vi "超标留样数据插入.vi"(0 "data输出":T1={"时间"=timestamp(3687928779.282504 s since 1904-01-01), "留样参数"="NH3N超标,超标浓度为0.000\r\n留样瓶号:0", "留样瓶号"=0.0}, 3 "错误输入（无错误）":errorcluster) -> (10 "错误输出":errorcluster)   [LabVIEW 2016]
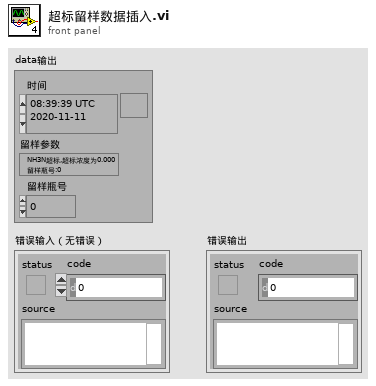
[diagram p1: front panel]
types:
  T1 = cluster{"时间":timestamp, "留样参数":string, "留样瓶号":dbl}
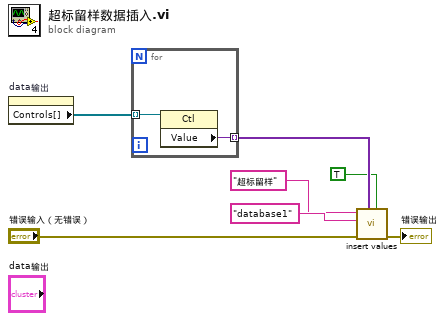
[diagram p0: block diagram]
diagram:
  n1 = property on="data输出" class="Clust (严格)"() -> ("Controls[]"=w1:refnum<vi>[])  [unwired: 2 in, 2 out]
  n2 = for {
    tunnel: w1 -> [w9] mode=indexing
    tunnel: [w8] -> w7 mode=indexing
    n3 = property class="Ctl"(reference=w9) -> ("Value"=w8:variant)  [unwired: 1 in, 2 out]
  }
  n4 = call "insert values.vi"("是否创建唯一键"=TRUE, "data"=w7, "错误输入（无错误）"="错误输入（无错误）", "database"="database1", "Tabe Name"="超标留样") -> ("错误输出"=→"错误输出":errorcluster)  [unwired: 6 in]
